vi "STM Write Meta Data (Serial Clst).vi"(6 "Options":T3={"Ignore Timeout Error"=TRUE, "timeout ms (1000)"=1000}, 7 "Meta data":T2[](array[typedef]), 8 "error in":errorcluster, 11 "Connection Info In":T1) -> (0 "error out":errorcluster, 3 "Connection Info Out":T1)   [LabVIEW 2014, in "QwaveSys Raspberry Pi Library.lvlib"]
doc: "Use this VI to transmit the meta data cluster to a remote computer. Sending the meta data to another computer helps maintainability since the data resides only on one side and it is shared to other computers at run time."
uses:
  QwaveSys Raspberry Pi Library.lvlib
  stm_Serial Connection Info.ctl
  _SubVIs/stm_MetaDataElement.ctl
  stm_Serial Write Options.ctl
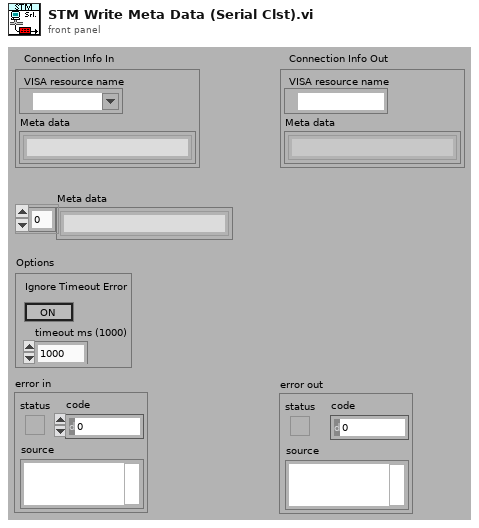
[diagram p1: front panel]
types:
  T1 = typedef "QwaveSys Raspberry Pi Library.lvlib/stm_Serial Connection Info.ctl" = cluster{"VISA resource name":refnum<visa-resource-name>, "Meta data":T2[]}
  T2 = typedef "QwaveSys Raspberry Pi Library.lvlib/stm_MetaDataElement.ctl" = string
  T3 = typedef "QwaveSys Raspberry Pi Library.lvlib/stm_Serial Write Options.ctl" = cluster{"Ignore Timeout Error":bool, "timeout ms (1000)":u32}
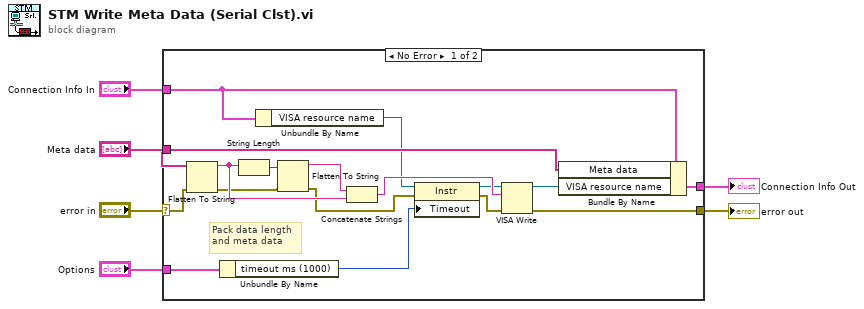
[diagram p0: block diagram]
diagram:
  n1 = case shown="No Error" "error in" {
    selector: "error in" -> [w14 w25]
    tunnel: [w16 w24] -> w6
    tunnel: "Connection Info In" -> [w12 w24]
    tunnel: "Meta data" -> [w15 _]
    tunnel: [w23 w25] -> w4
    tunnel: "Options" -> [w18 _]
    frame No Error {
      # "Pack data length\nand meta data"
      n2 = Flatten To String(anything=w15, error in (no error)=w14) -> (data string=w19:string, error out=w13:errorcluster)  [unwired: 3 out]
      n3 = Unbundle By Name(w18) -> ("timeout ms (1000)"=w9:u32)
      n4 = String Length(string=w19) -> (length=w22:i32)
      n5 = Unbundle By Name(w12) -> ("VISA resource name"=w11:refnum<visa-resource-name>)
      n6 = Flatten To String(anything=w22, error in (no error)=w13) -> (data string=w21:string, error out=w8:errorcluster)  [unwired: 3 out]
      n7 = Concatenate Strings(w21, w19) -> (w20:string)
      n8 = property class="Instr"(reference=w11, error in=w8, "Timeout"=w9) -> (reference out=w10:refnum<visa-resource-name>, error out=w7:errorcluster)
      n9 = VISA Write(VISA resource name=w10, write buffer=w20, error in (no error)=w7) -> (VISA resource name out=w17:refnum<visa-resource-name>, error out=w23:errorcluster)  [unwired: 1 out]
      n10 = Bundle By Name(cluster=w12, "Meta data"=w15, "VISA resource name"=w17) -> (w16:T1)
    }
    frame Error {
    }
  }
  "Connection Info Out" <- w6
  "error out" <- w4
